vi "DAQ_Digital Pulse Gen Initialize.vi"(0 "Physical Channel (Counter)":tag, 1 "Output Terminal":tag, 7 "Global Channel (counter)":refnum<k21>, 11 "error in":errorcluster) -> (4 "DAQmx Task Out":refnum<k21>, 15 "error out":errorcluster)   [LabVIEW 2021, in "DAQ_Digital Pulse Generation.lvlib"]
doc: "Initialize counter output channel and obtains a DAQmx task. Get Physical/Global channel of counter and output terminal to generate.\n\nNote: Multiple counters cannot be initialized in the same task. Use a separate task for each counter."
uses:
  DAQ_Digital Pulse Generation.lvlib
  <vilib>/DAQmx/create/channels.llb/DAQmx Create Channel (CO-Pulse Generation-Time).vi
  <resource>/objmgr/daqmx.rc
panel:
  # "Inputs"
  # "Outputs"
  # "Overview:\nThis VI initializes the counter of DIO Module for Digital Pulse Generation and provides the DAQmx Task Out\n\nHardware Requirement: A compatible PXI, PCIe, USB, cDAQ or Testscale device\n\nSoftware Requirement: NI DAQmx 2022 Q4 or later\n\nInstructions:\n1. Enter physical channel of counter to use for Digital pulse generation in Physical Channel (Counter) control. (Or) Enter Global channel to use instead of initiating a new task. User must configure only one input. If both are provided, Global Channels will take precedence.\n2. Enter Output Terminal on which the signal to be measured. Refer Help for more details on the default terminals of each counters. User can configure different PFI lines as well. \n3. Get the Digital Pulse Generation task from DAQmx Task Out\n\nNotes: \n1. User can use the DAQmx Task on other VIs to configure and initiate Digital Pulse Generation.\n2. Multiple counters cannot be initialized in the same task. Use a separate task for each counter."
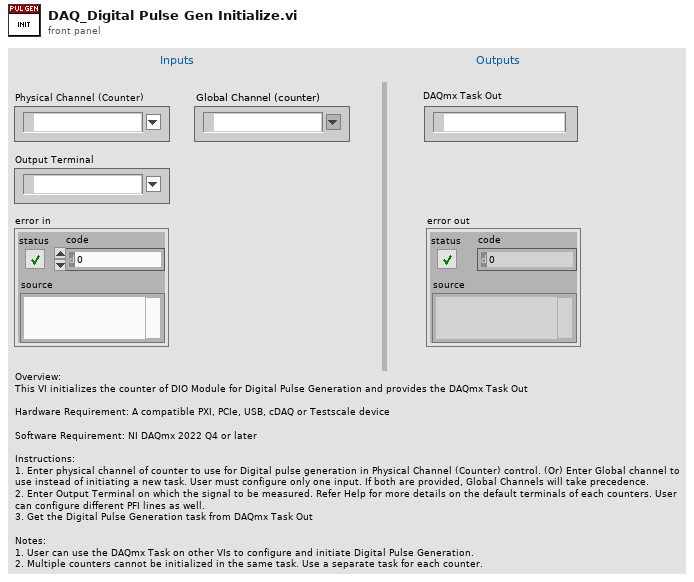
[diagram p1: front panel]
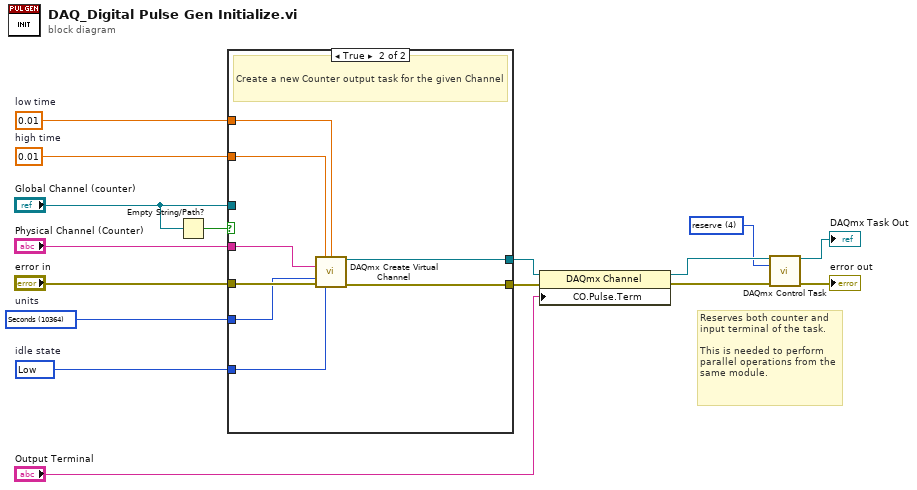
[diagram p0: block diagram]
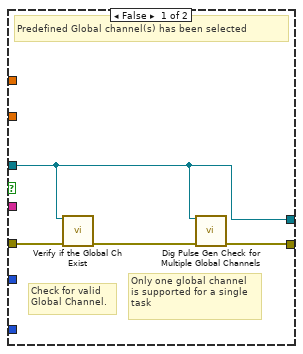
[diagram p2: hidden frame]
diagram:
  w3 = 0.01  # high time
  w4 = 0.01  # low time
  w5 = 10364 items=["Seconds"=10364]  # units
  w6 = 10214 items=["High"=10192, "Low"=10214]  # idle state
  w7 = 4 items=["verify"=2, "reserve"=4, "commit"=3, "unreserve"=5, "abort"=6] ("action")
  # "Reserves both counter and input terminal of the task.\n\nThis is needed to perform parallel operations from the same module."
  n1 = Empty String/Path?(string/path="Global Channel (counter)") -> (empty?=w2:bool)
  n2 = case shown="True" w2 {
    tunnel: "error in" -> [w19 w28]
    tunnel: [w17 w27] -> w15
    tunnel: "Physical Channel (Counter)" -> [_ w26]
    tunnel: [w18 w25] -> w12
    tunnel: w6 -> [_ w24]
    tunnel: w5 -> [_ w23]
    tunnel: w4 -> [_ w22]
    tunnel: w3 -> [_ w21]
    tunnel: "Global Channel (counter)" -> [w18 _]
    frame False {
      # "Only one global channel\nis supported for a single\ntask"
      # "Check for valid \nGlobal Channel."
      # "Predefined Global channel(s) has been selected"
      n3 = call "Verify if the Global Ch Exist.vi"("Global Channels"=w18, "error in (no error)"=w19) -> ("error out"=w20:errorcluster)  [unwired: 13 in]
      n4 = call "Dig Pulse Gen Check for Multiple Global Channels.vi"("Global Channel In"=w18, "error in (no error)"=w20) -> ("error out"=w17:errorcluster)  [unwired: 12 in, 1 out]
    }
    frame True {
      # "Create a new Counter output task for the given Channel"
      n5 = call-poly <vilib>:"DAQmx Create Virtual Channel.vi"("high time"=w21, "low time"=w22, "counter"=w26, "units"=w23, "error in"=w28, "idle state"=w24) -> ("task out"=w25:refnum<k21>, "error out"=w27:errorcluster)  [unwired: 8 in]
    }
  }
  n6 = property class="DAQmx Channel"(reference=w12, error in=w15, "CO.Pulse.Term"="Output Terminal") -> (reference out=w9:refnum<k21>, error out=w13:errorcluster)
  n7 = call <vilib>:"DAQmx Control Task.vi"("task/channels in"=w9, "action"=w7, "error in"=w13) -> ("task out"=→"DAQmx Task Out":refnum<k21>, "error out"=→"error out":errorcluster)  [unwired: 11 in]
